vi "Close.vi"(8 "error in (no error)":errorcluster, 11 "uService Template in":refnum<class "Detector Manager.lvclass">) -> (0 "error out":errorcluster, 3 "uService Template out":refnum<class "Detector Manager.lvclass">)   [LabVIEW 2026, in "TALOS.lvlib" / "Detector Manager.lvlib" / "Detector Manager.lvclass"]
uses:
  Detector Manager.lvclass
  Detector Manager.lvclass/Detector Manager.ctl
  Father of all uServices/Father of all uServices/Father of all uServices.lvclass
  Classes/Father of all Detectors/Father Of All Detectors.lvclass
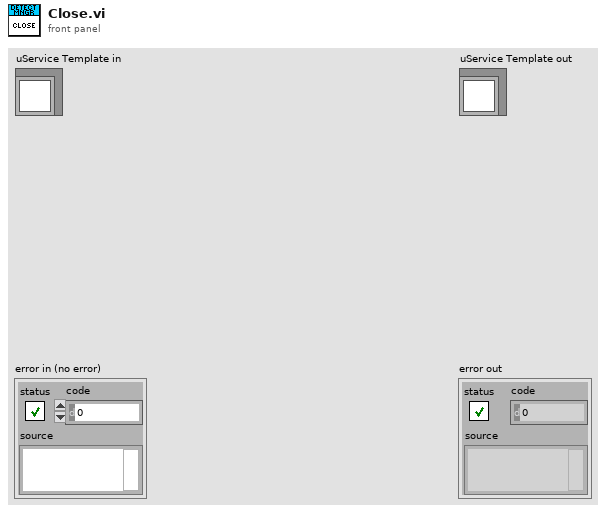
[diagram p1: front panel]
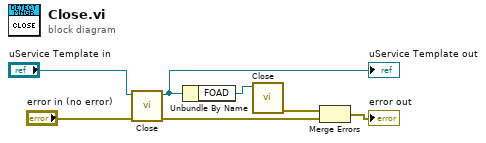
[diagram p0: block diagram]
diagram:
  n1 = call-parent "Close.vi"("error in (no error)"="error in (no error)", "uService Template in"="uService Template in") -> ("error out"=w7:errorcluster, "uService Template out"=w4:refnum<class "Detector Manager.lvclass">)  [unwired: 8 in]
  "uService Template out" <- w4
  n2 = Unbundle By Name(w4) -> ("FOAD"=w3:refnum<class "Father Of All Detectors.lvclass">)
  n3 = call-dynamic "Close.vi"("Father Of All Detectors in"=w3) -> ("error out"=w1:errorcluster)  [unwired: 9 in, 1 out]
  n4 = Merge Errors(w1, w7) -> (→"error out":errorcluster)
